vi "fix_negative_zero.vi"(1 "String IN":string) -> (0 "String OUT":string)   [LabVIEW 2019]
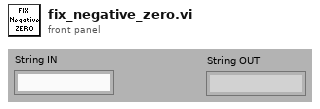
[diagram p1: front panel]
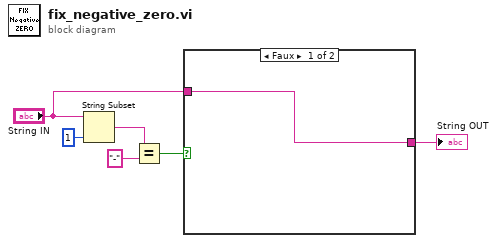
[diagram p0: block diagram]
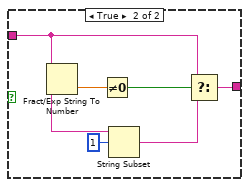
[diagram p2: hidden frame]
diagram:
  n1 = String Subset(string="String IN", length (rest)=1 ("length (rest)")) -> (substring=w3:string)  [unwired: 1 in]
  n2 = Equal?(x=w3, y="-") -> (x = y?=w4:bool)
  n3 = case shown="Faux" w4 {
    tunnel: "String IN" -> [w7 w9]
    tunnel: [w7 w8] -> w1
    frame False {
    }
    frame True {
      n4 = Fract/Exp String To Number(string=w9) -> (number=w13:dbl)  [unwired: 3 in, 1 out]
      n5 = Not Equal To 0?(x=w13) -> (x != 0?=w12:bool)
      n6 = String Subset(string=w9, offset (0)=1) -> (substring=w10:string)  [unwired: 1 in]
      n7 = Select(t=w9, s=w12, f=w10) -> (s? t:f=w8:string)
    }
  }
  "String OUT" <- w1
